vi "read meter (high level).vi"(7 "beep (off)":bool, 8 "previous values":T1 {"time (s)" format="%.2f"; "temperature" format="%.2f"; "channel 2" format="%.2f"; "channel 1" format="%.2f"}, 9 "seconds/data point":u16, 10 "2nd channel":bool, 11 "Serial Port":refnum<visa-resource-name>) -> (0 "current values":T1 {"time (s)" format="%.2f"; "temperature" format="%.2f"; "channel 2" format="%.3f"; "channel 1" format="%.3f"}, 1 "units B":string, 2 "units A":string, 3 "Sample ID":u16, 4 "new data":ext[](array[numeric]), 5 "got data":bool)   [LabVIEW 2010]
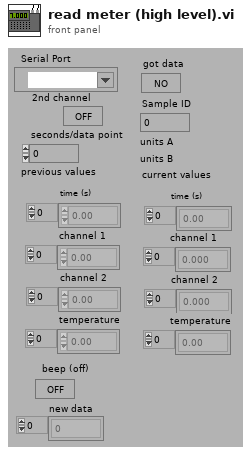
[diagram p1: front panel]
types:
  T1 = cluster{"channel 1":dbl[], "channel 2":dbl[], "temperature":dbl[], "time (s)":sgl[]}
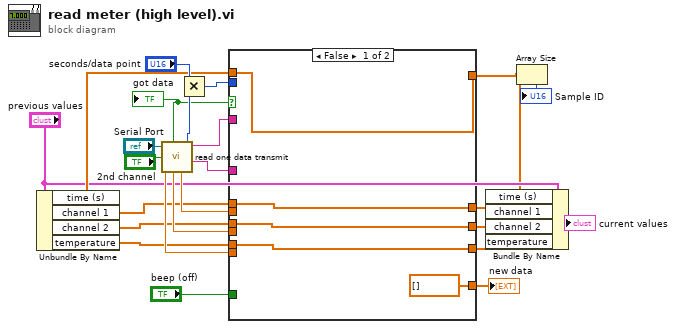
[diagram p0: block diagram]
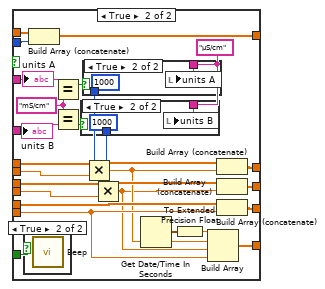
[diagram p2: hidden frame]
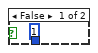
[diagram p3: hidden frame]
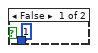
[diagram p4: hidden frame]
diagram:
  n1 = Unbundle By Name("previous values") -> ("time (s)"=w13:sgl[], "channel 1"=w12:dbl[], "channel 2"=w11:dbl[], "temperature"=w10:dbl[])
  n2 = call "read one data transmit.vi"("Serial Port"="Serial Port", "2nd channel"="2nd channel") -> ("got data"=w2:bool, "Temperature"=w15:sgl, "Channel 2"=w23:sgl, "Sample ID"=w19:u32, "Channel 1 units"=w21:string, "Channel 1"=w24:sgl, "Channel 2 units"=w20:string)  [unwired: 2 out]
  "got data" <- w2
  n3 = Multiply(x="seconds/data point", y=w19) -> (x*y=w22:u32)
  n4 = case shown="False" w2 {
    tunnel: [w27 w55] -> w4
    tunnel: [w28 w54] -> w5
    tunnel: [w29 w53] -> w6
    tunnel: w10 -> [w27 w52]
    tunnel: w11 -> [w28 w51]
    tunnel: w12 -> [w29 w50]
    tunnel: w15 -> [_ w35]
    tunnel: w23 -> [_ w49]
    tunnel: w24 -> [_ w48]
    tunnel: w13 -> [w26 w47]
    tunnel: [w26 w46] -> w7
    tunnel: w22 -> [_ w45]
    tunnel: w21 -> [_ w44]
    tunnel: w20 -> [_ w41]
    tunnel: "beep (off)" -> [_ w43]
    tunnel: [ext[] [] w30] -> w1
    frame False {
    }
    frame True {
      w36 = "µS/cm"
      w42 = "mS/cm"
      n5 = case shown="True" w43 {
        frame False {
        }
        frame True {
          n6 = call <vilib>:"Beep.vi"() -> ()  [unwired: 12 in]
        }
      }
      n7 = Build Array (concatenate)(w47, w45) -> (w46:sgl[])
      n8 = Equal?(x=w44, y=w42) -> (x = y?=w40:bool)
      n9 = Equal?(x=w42, y=w41) -> (x = y?=w38:bool)
      n10 = case shown="True" w38 {
        tunnel: [1 1000] -> w37
        tunnel: w36 -> [_ w57]
        frame False {
        }
        frame True {
          n11 = local write "units B"(w57) -> ()
        }
      }
      n12 = case shown="True" w40 {
        tunnel: [1 1000] -> w39
        tunnel: w36 -> [_ w60]
        frame False {
        }
        frame True {
          n13 = local write "units A"(w60) -> ()
        }
      }
      n14 = Multiply(x=w39, y=w48) -> (x*y=w34:sgl)
      n15 = Multiply(x=w37, y=w49) -> (x*y=w33:sgl)
      n16 = Get Date/Time In Seconds() -> (seconds since 1Jan1904=w31:timestamp)
      n17 = To Extended Precision Float(1:w31) -> (0:w32:ext)
      n18 = Build Array(w32, w34, w33, w35) -> (w30:ext[])
      n19 = Build Array (concatenate)(w50, w34) -> (w53:dbl[])
      n20 = Build Array (concatenate)(w51, w33) -> (w54:dbl[])
      n21 = Build Array (concatenate)(w52, w35) -> (w55:dbl[])
      "units B" <- w41
      "units A" <- w44
    }
  }
  "new data" <- w1
  n22 = Bundle By Name(cluster="previous values", "time (s)"=w7, "channel 1"=w6, "channel 2"=w5, "temperature"=w4) -> (→"current values":T1)
  n23 = Array Size(array=w7) -> (size(s)=→"Sample ID":i32)
